vi "Parse Spectra Data.vi"() -> ()   [LabVIEW 2016]
panel:
  out "Re-starts 2":timestamp[](array[timestamp])
  out "Waveform Graph":dbl[](graph)
  out "Array - String":string[](array[string])
  in  "m file":path=path "\\\\eden\\NHMFLDATA/Data/RUS, JEvans/8-6-2018, Annealing RUS of JE-AlRPR-1, Second Try, RAW DATA/080618/m001_080618.tdms"
  out "Re-starts":timestamp[](array[timestamp])
  in  "RUS Log path":path=path "\\\\eden\\NHMFLDATA/Data/RUS, JEvans/8-6-2018, Annealing RUS of JE-AlRPR-1, Second Try, RAW DATA/RUS Log.txt"
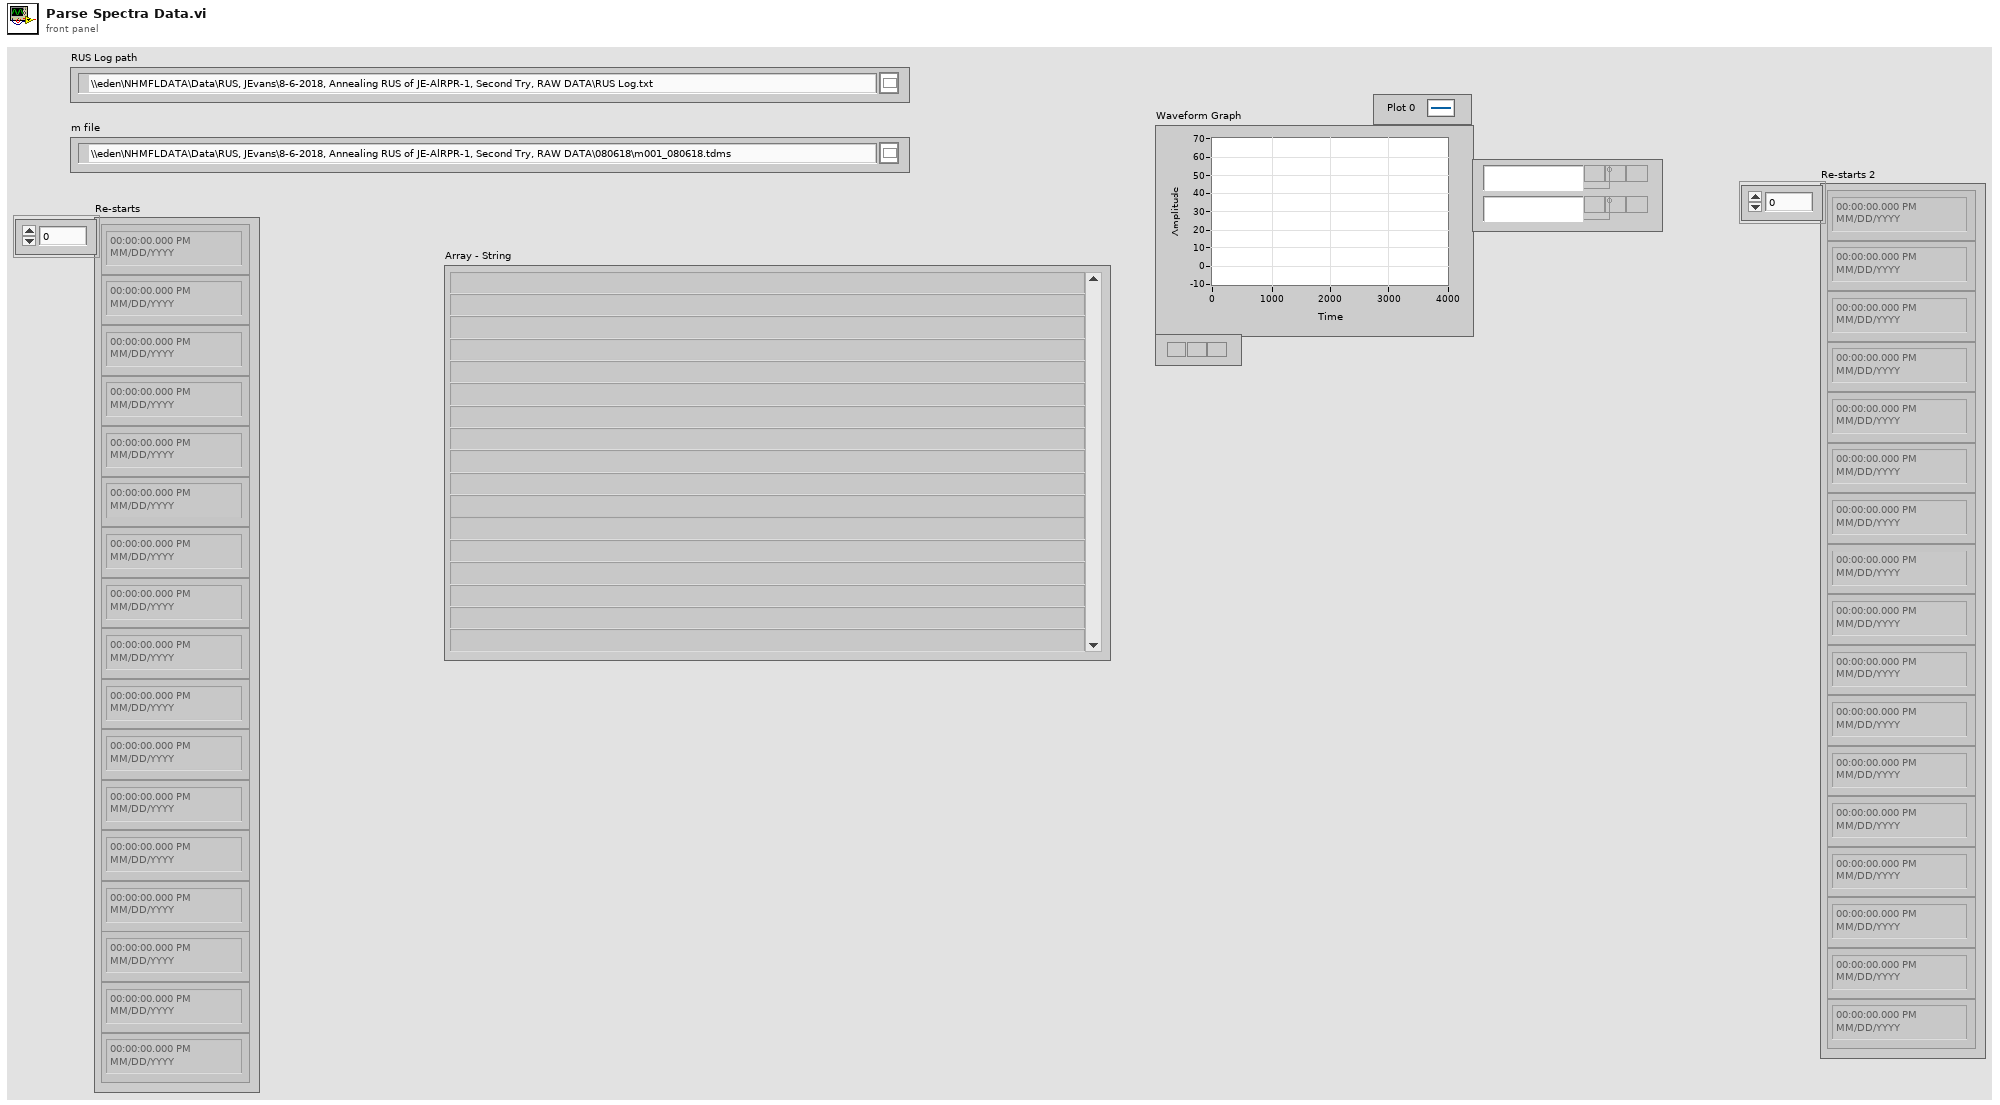
[diagram p1: front panel]
types:
  T1 = enum16{"open", "open or create", "create or replace", "create", "open (read-only)"}
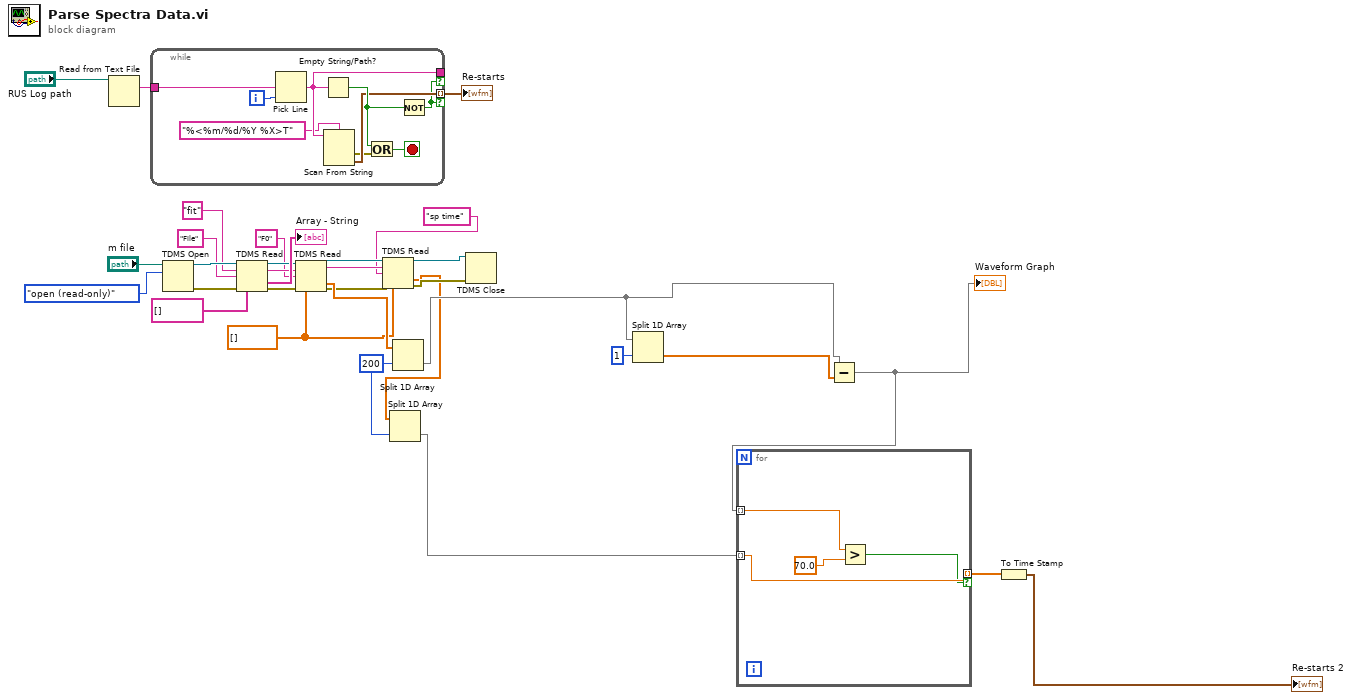
[diagram p0: block diagram]
diagram:
  w6 = 200 ("index")
  w7 = dbl[] []
  n1 = Read from Text File(file (use dialog)="RUS Log path") -> (text=w31:string)  [unwired: 3 in, 3 out]
  n2 = while {
    tunnel: w31 -> [w41]
    tunnel: [w39] -> _ if=w36
    tunnel: [w37] -> w30 mode=indexing if=w36
    i -> [w35]
    stop <- w34 stop-if-true
    n3 = Pick Line(multi-line string=w41, line index=w35) -> (output string=w39:string)  [unwired: 1 in]
    n4 = Empty String/Path?(string/path=w39) -> (empty?=w40:bool)
    n5 = Scan From String(format string="%<%m/%d/%Y %X>T", input string=w39) -> (error out=w33:errorcluster, output 1=w37:timestamp)  [unwired: 3 in, 2 out]
    n6 = Or(x=w40, y=w33) -> (x .or. y?=w34:bool)
    n7 = Not(x=w40) -> (.not. x?=w36:bool)
  }
  "Re-starts" <- w30
  n8 = TDMS Open(10:T1."open (read-only)" ("operation (0:open)"), 11:"m file") -> (0:w26:errorcluster, 3:w27:refnum<k34>)  [unwired: 5 in]
  n9 = TDMS Read(0:w27, 5:"fit" ("group name in"), 7:"File", 11:w26, 12:string[] []) -> (4:w20:refnum<k34>, 6:w19:string, 10:→"Array - String":string[], 15:w21:errorcluster)  [unwired: 3 in, 2 out]
  n10 = TDMS Read(0:w20, 5:w19, 7:"F0", 11:w21, 12:w7) -> (4:w12:refnum<k34>, 6:w9:string, 10:w15:dbl[], 15:w13:errorcluster)  [unwired: 3 in, 2 out]
  n11 = TDMS Read(0:w12, 5:w9, 7:"sp time", 11:w13, 12:w7) -> (4:w10:refnum<k34>, 10:w5:dbl[], 15:w11:errorcluster)  [unwired: 3 in, 3 out]
  n12 = Split 1D Array(array=w5, index=w6) -> (second subarray=w3:dbl[])  [unwired: 1 out]
  n13 = Split 1D Array(array=w15, index=w6) -> (second subarray=w14:dbl[])  [unwired: 1 out]
  n14 = TDMS Close(8:w11, 11:w10) -> ()  [unwired: 2 out]
  n15 = Split 1D Array(array=w14, index=1) -> (second subarray=w16:dbl[])  [unwired: 1 out]
  n16 = Subtract(x=w14, y=w16) -> (x-y=w4:dbl[])
  "Waveform Graph" <- w4
  n17 = for {
    tunnel: w4 -> [w45] mode=indexing
    tunnel: w3 -> [w43] mode=indexing
    tunnel: [w43] -> w2 mode=indexing if=w42
    n18 = Greater?(x=w45, y=70.0) -> (0:w42:bool)
  }
  n19 = To Time Stamp(1:w2) -> (0:→"Re-starts 2":timestamp[])
